vi "Keithley 3940 test ramp.vi"   [LabVIEW 2025]
doc: "Author: Scott Hannahs <sth@magnet.fsu.edu>\n\nThis software is licensed for use under the “MIT License\"\nCopyright (c) 2025 Scott Hannahs, sth@sth@magnet.sthnet.net\n\nPermission is hereby granted, free of charge, to any person obtaining a copy of this software and associated documentation files (the \"Software\"), to deal in the Software without restriction, including without limitation the rights to use, copy, modify, merge, publish, distribute, sublicense, and/or sell copies of the Software, and to permit persons to whom the Software is furnished to do so, subject to the following conditions: The above copyright notice and this permission notice shall be included in all copies or substantial portions of the Software.\n\nTHE SOFTWARE IS PROVIDED \"AS IS\", WITHOUT WARRANTY OF ANY KIND, EXPRESS OR IMPLIED, INCLUDING BUT NOT LIMITED TO THE WARRANTIES OF MERCHANTABILITY, FITNESS FOR A PARTICULAR PURPOSE AND NONINFRINGEMENT. IN NO EVENT SHALL THE AUTHORS OR COPYRIGHT HOLDERS BE LIABLE FOR ANY CLAIM, DAMAGES OR OTHER LIABILITY, WHETHER IN AN ACTION OF CONTRACT, TORT OR OTHERWISE, ARISING FROM, OUT OF OR IN CONNECTION WITH THE SOFTWARE OR THE USE OR OTHER DEALINGS IN THE SOFTWARE."
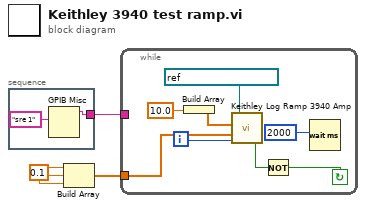
[diagram p0: block diagram]
diagram:
  w2 = 0.1
  n1 = stacked-sequence {
    tunnel: [w4] -> w3
    frame #0 {
      n2 = GPIB Misc(0:"sre 1") -> (2:w4:string)  [unwired: 1 in, 2 out]
    }
  }
  n3 = Build Array(w2, w2, w2) -> (w1:dbl[])
  n4 = while {
    tunnel: w1 -> [w6]
    tunnel: w3 -> [_]
    i -> [w9]
    stop <- w8 continue-if-true
    n5 = Build Array(10.0) -> (w10:dbl[])
    n6 = call "Keithley Log Ramp 3940 Amp.vi"("Point #"=w9, "GPIB Data In"=w6, "Parameters"=w10, "VISA session"=refnum<visa-resource-name> "GPIB0::2::INSTR") -> ("Stop"=w7:bool)  [unwired: 1 out]
    n7 = Not(x=w7) -> (.not. x?=w8:bool)
    n8 = Wait (ms)(milliseconds to wait=2000) -> ()  [unwired: 1 out]
  }
